vi "Read can loop.vi"(7 "Signals For Conversion":string[](array[string]), 8 "error in (no error)":errorcluster, 9 "Numeric":i32, 10 "tdms file in":refnum<k34>, 11 "Frame Signal Conversion in":refnum<class "Frame Signal Conversion.lvclass">) -> (0 "error out":errorcluster, 1 "Error and warning map":map{string, i8}(c390), 2 "Signal map":map{string, dbl}(c390), 3 "tdms file out":refnum<k34>)   [LabVIEW 2024]
uses:
  PROD_LabView_Libraries/PCAN-XNET/PCan_Xnet.lvlib
  <instrlib>/KDI Digital Instrumentation/API_for_PCAN_BASIC_FD/TPCANHandle.ctl
  PROD_LabView_Libraries/Frame signal conversion/Frame Signal Conversion Version 8/Frame Signal Conversion.lvclass
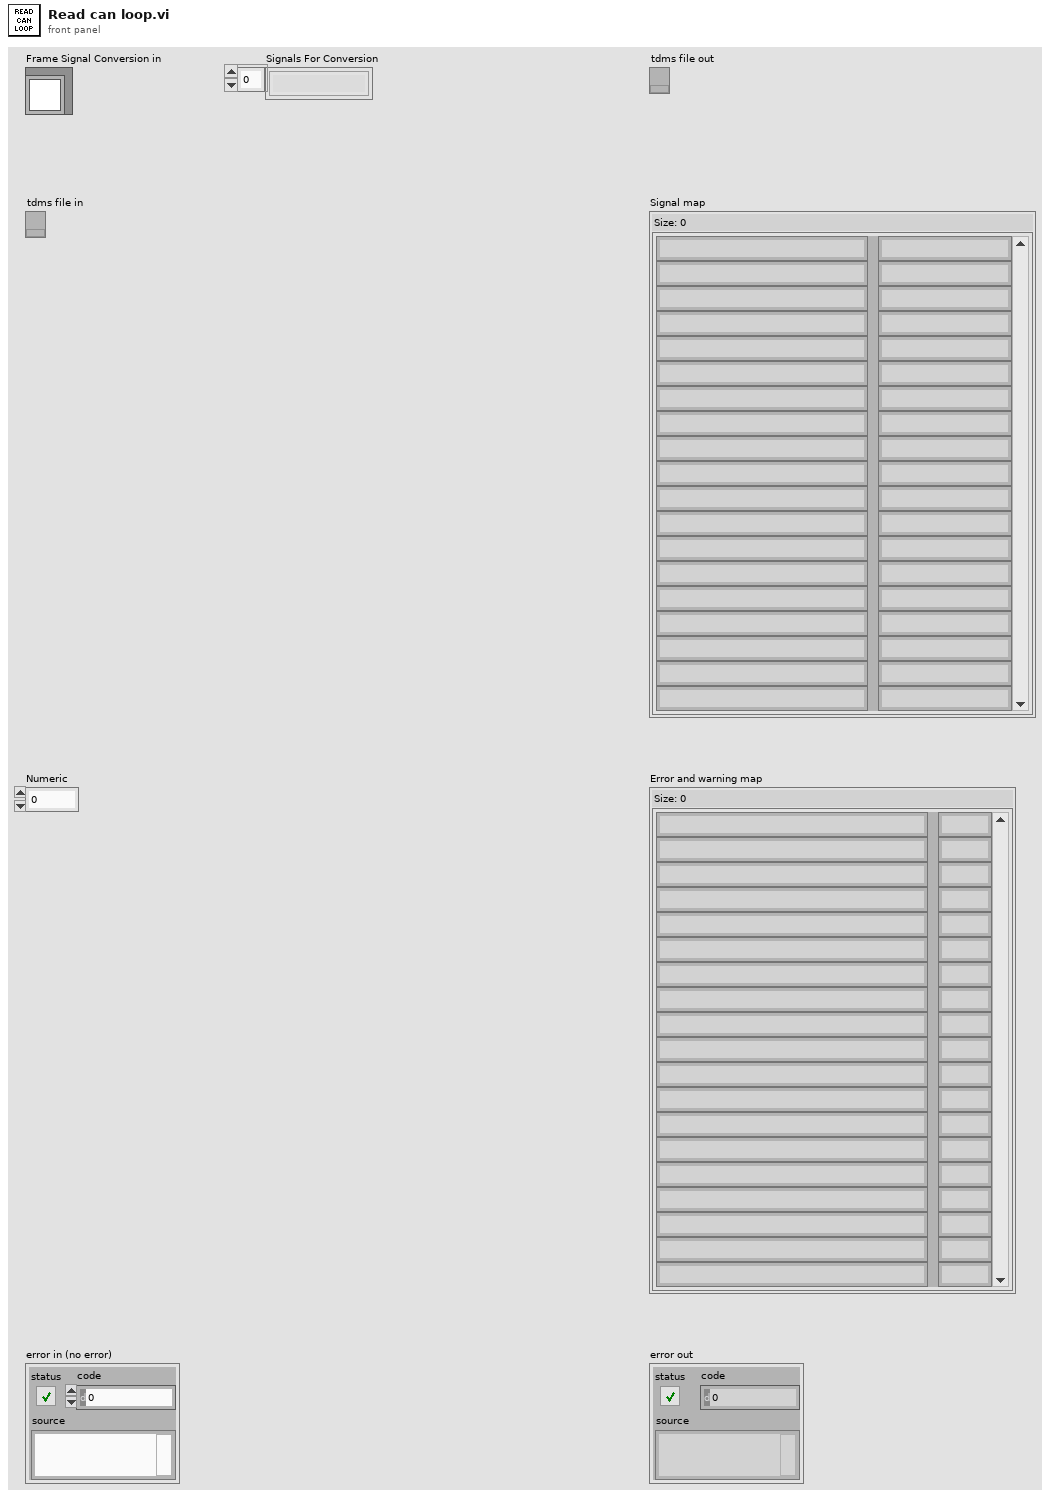
[diagram p1: front panel]
types:
  T1 = typedef "TPCANHandle.ctl" = enum16{"PCAN_NONEBUS  0x000", "PCAN_ISABUS1  0x21", "PCAN_ISABUS2  0x22", "PCAN_ISABUS3  0x23", "PCAN_ISABUS4  0x24", "PCAN_ISABUS5  0x25", "PCAN_ISABUS6  0x26", "PCAN_ISABUS7  0x27", "PCAN_ISABUS8  0x28", "PCAN_DNGBUS1  0x31", "PCAN_PCIBUS1  0x41", "PCAN_PCIBUS1  0x42", "PCAN_PCIBUS1  0x43", "PCAN_PCIBUS1  0x44", "PCAN_PCIBUS1  0x45", "PCAN_PCIBUS1  0x46", "PCAN_PCIBUS1  0x47", "PCAN_PCIBUS1  0x48", "PCAN_PCIBUS1  0x409", "PCAN_PCIBUS1  0x40A", "PCAN_PCIBUS1  0x40B", "PCAN_PCIBUS1  0x40C", "PCAN_PCIBUS1  0x40D", "PCAN_PCIBUS1  0x40E", "PCAN_PCIBUS1  0x40F", "PCAN_PCIBUS1  0x410", "PCAN_USBBUS1  0x51", "PCAN_USBBUS2  0x52", "PCAN_USBBUS3  0x53", "PCAN_USBBUS4  0x54", "PCAN_USBBUS5  0x55", "PCAN_USBBUS6  0x56", "PCAN_USBBUS7  0x57", "PCAN_USBBUS8  0x58", "PCAN_USBBUS9  0x509", "PCAN_USBBUS10  0x50A", "PCAN_USBBUS11  0x50B", "PCAN_USBBUS12  0x50C", "PCAN_USBBUS13  0x50D", "PCAN_USBBUS14  0x50E", "PCAN_USBBUS15  0x50F", "PCAN_USBBUS16  0x510", "PCAN_PCCBUS1  0x61", "PCAN_PCCBUS2  0x62", "PCAN_LANBUS1  0x801", "PCAN_LANBUS2  0x802", "PCAN_LANBUS3  0x803", "PCAN_LANBUS4  0x804", "PCAN_LANBUS5  0x805", "PCAN_LANBUS6  0x806", "PCAN_LANBUS7  0x807", "PCAN_LANBUS8  0x808", "PCAN_LANBUS9  0x809", "PCAN_LANBUS10  0x80A", "PCAN_LANBUS11  0x80B", "PCAN_LANBUS12  0x80C", "PCAN_LANBUS13  0x80D", "PCAN_LANBUS14  0x80E", "PCAN_LANBUS15  0x80F", "PCAN_LANBUS16  0x810"}
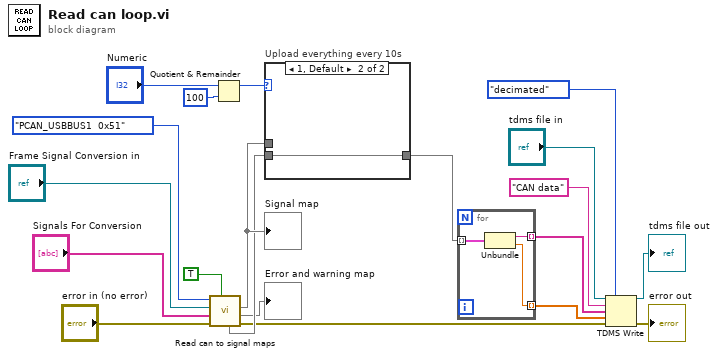
[diagram p0: block diagram]
diagram:
  n1 = call "Read can to signal maps.vi"("Run once"=TRUE, "error in (no error)"="error in (no error)", "Signals For Conversion"="Signals For Conversion", "Frame signal conversion.lvlib:Frame Signal Conversion.lvclass"="Frame Signal Conversion in", "TPCANHandle"=TPCANHandle."PCAN_USBBUS1  0x51") -> ("error out"=w8:errorcluster, "Error and warning map"=→"Error and warning map":map{string, i8}, "Signal map"=w20:map{string, dbl}, "New data"=w11:map{string, dbl})  [unwired: 3 in]
  "Signal map" <- w20
  n2 = Quotient & Remainder(x="Numeric", y=100) -> (x-y*floor(x/y)=w18:i32)  [unwired: 1 out]
  n3 = case "Upload everything every 10s" shown="1, Default" w18 {
    tunnel: w20 -> [w21 _]
    tunnel: w11 -> [_ w22]
    tunnel: [w21 w22] -> w17
    frame 0 {
    }
    frame 1, Default {
    }
  }
  n4 = for {
    tunnel: w17 -> [w25] mode=indexing
    tunnel: [w23] -> w13 mode=indexing
    tunnel: [w24] -> w14 mode=indexing
    n5 = Unbundle(w25) -> (w23:string, w24:dbl)
  }
  n6 = TDMS Write(0:"tdms file in", 1:enum16{"decimated", "interleaved"}."decimated" ("data layout (0:decimated)"), 5:"CAN data" ("group name in (Untitled)"), 7:w13, 9:w14, 11:w8) -> (4:→"tdms file out":refnum<k34>, 15:→"error out":errorcluster)  [unwired: 2 out]
